vi "Plot Data and Print.vi"(0 "File:":string, 4 "x axis column":i32, 5 "Data":dbl[][](array[numeric]) format="%.2e", 6 "Col heading":string[](array[string]), 7 "Display/hide":bool[](array[boolean]), 8 "Print":bool, 9 "Index":i32) -> (3 "Data Plot":cluster{dbl[], dbl[]}[](graph))   [LabVIEW 2021]
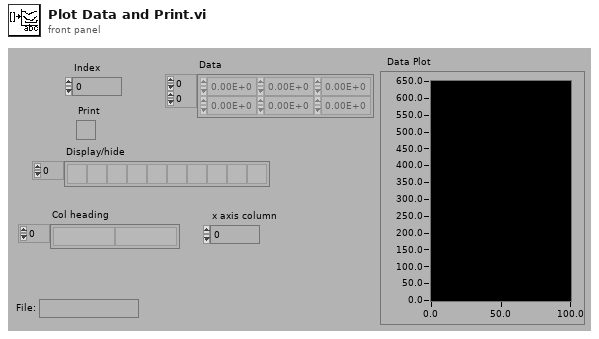
[diagram p1: front panel]
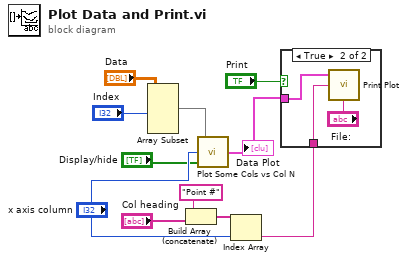
[diagram p0: block diagram]
diagram:
  n1 = Array Subset(array="Data", length (row)="Index") -> (w5:dbl[][])  [unwired: 3 in]
  n2 = Build Array (concatenate)("Point #", "Col heading") -> (w10:string[])
  n3 = call "Plot Some Cols vs Col N.vi"("Display/hide"="Display/hide", "Column for abscissa"="x axis column", "Input Array"=w5) -> ("Output Graph"=w1:cluster{dbl[], dbl[]}[])
  "Data Plot" <- w1
  n4 = Index Array(array=w10, index="x axis column") -> (element=w8:string)
  n5 = case shown="True" "Print" {
    tunnel: w8 -> [_ w13]
    tunnel: w1 -> [_ w12]
    frame False {
    }
    frame True {
      n6 = call "Print Plot.vi"("File:"="File:", "X-Axis Label"=w13, "Data Plot"=w12) -> ()
    }
  }
